vi "TimeSyncServ_GetAll.vi"() -> (0 "PV_TimeSyncStopServ":bool, 1 "PV_TimeSyncLastSentTime":i64, 2 "PV_TimeSyncLastRcvTim":i64, 3 "PV_TimeSyncLastRcvId":i8, 4 "PV_TimeSyncLoopCount":i32, 5 "PV_TimeSyncLastRcvVer":i8)   [LabVIEW 2019, in "PhotonVisionLib.lvlib"]
doc: "Get information on photonvision time sync server.\n\nInputs:\n - <None>\n\nOutputs:"
uses:
  PhotonVisionLib.lvlib
  PhotonVision_Globals.vi
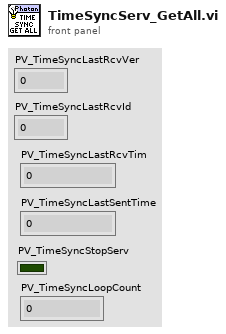
[diagram p1: front panel]
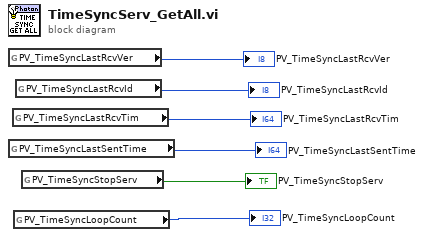
[diagram p0: block diagram]
diagram:
  n1 = global read "PhotonVision_Globals.vi" "PV_TimeSyncLastRcvVer"() -> (→"PV_TimeSyncLastRcvVer":i8)
  n2 = global read "PhotonVision_Globals.vi" "PV_TimeSyncLastSentTime"() -> (→"PV_TimeSyncLastSentTime":i64)
  n3 = global read "PhotonVision_Globals.vi" "PV_TimeSyncLastRcvTim"() -> (→"PV_TimeSyncLastRcvTim":i64)
  n4 = global read "PhotonVision_Globals.vi" "PV_TimeSyncLoopCount"() -> (→"PV_TimeSyncLoopCount":i32)
  n5 = global read "PhotonVision_Globals.vi" "PV_TimeSyncLastRcvId"() -> (→"PV_TimeSyncLastRcvId":i8)
  n6 = global read "PhotonVision_Globals.vi" "PV_TimeSyncStopServ"() -> (→"PV_TimeSyncStopServ":bool)
